vi "Sort Header Types.vi"(8 "error in (no error)":errorcluster, 11 "request headers":cluster{"header":string, "value":string}[](array[cluster])) -> (0 "error out":errorcluster, 2 "Request Headers":cluster{"header":string, "value":string}[](array[cluster]), 3 "Content-Headers":cluster{"header":string, "value":string}[](array[cluster]))   [LabVIEW 2018, in "HttpClient_NET.lvlib" / "HttpRequestMessage.lvclass"]
doc: "<b> </b> <b> </b>\nHttpClient_NET\nJustin Young - Viviota\nCopyright (c) 2021\nLicense: BSD"
uses:
  HttpRequestMessage.lvclass
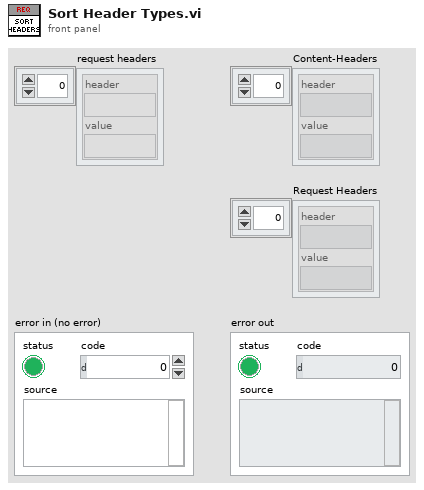
[diagram p1: front panel]
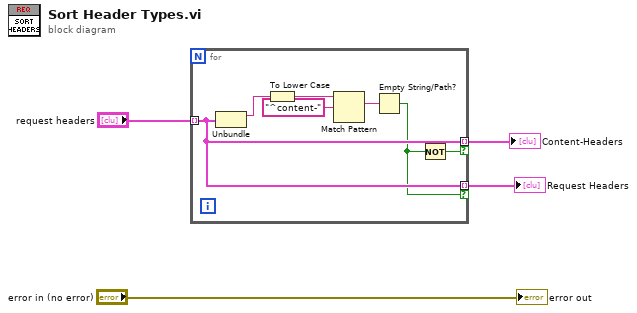
[diagram p0: block diagram]
diagram:
  n1 = for {
    tunnel: "request headers" -> [w7] mode=indexing
    tunnel: [w7] -> w3 mode=indexing if=w5
    tunnel: [w7] -> w2 mode=indexing if=w6
    n2 = Unbundle(w7) -> ("header"=w11:string)  [unwired: 1 out]
    n3 = To Lower Case(string=w11) -> (all lower case string=w10:string)
    n4 = Match Pattern(string=w10, regular expression="^content-") -> (match substring=w8:string)  [unwired: 1 in, 3 out]
    n5 = Empty String/Path?(string/path=w8) -> (empty?=w6:bool)
    n6 = Not(x=w6) -> (.not. x?=w5:bool)
  }
  "Content-Headers" <- w3
  "Request Headers" <- w2
  "error out" <- "error in (no error)"
